vi "deleteDesFromEEPROMFiles.vi"(11 "input_eeprom":string[][](array[string])) -> (3 "show_eeprom":string[][](array[string]))   [LabVIEW 2011]
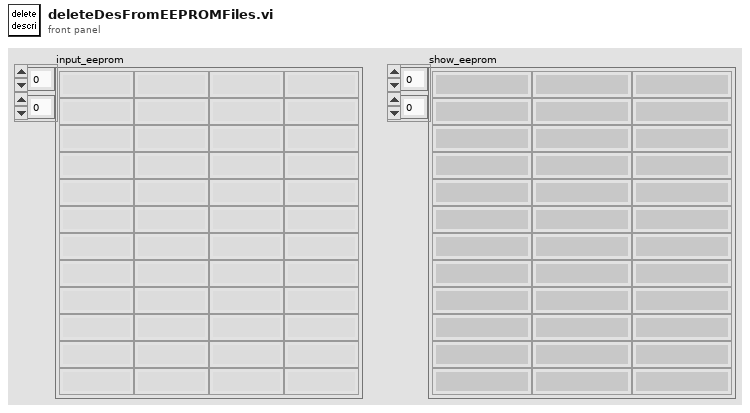
[diagram p1: front panel]
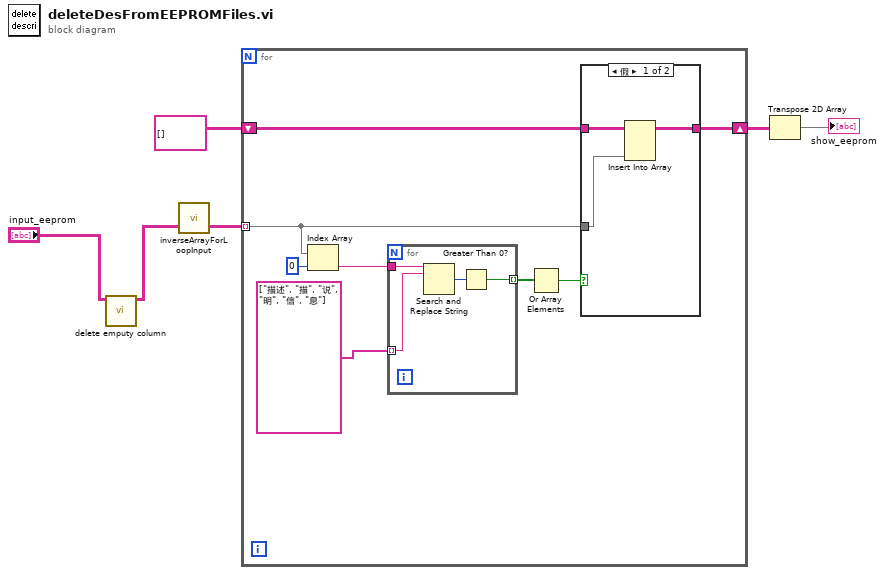
[diagram p0: block diagram]
diagram:
  n1 = call "delete emputy column.vi"("input_eeprom"="input_eeprom") -> ("input_eeprom_deleteemputycolumn"=w1:string[][])  [unwired: 10 in]
  n2 = call "inverseArrayForLoopInput.vi"("input_array_temp_str"=w1) -> ("show_array_temp_str"=w6:string[][])  [unwired: 1 in, 1 out]
  n3 = for {
    tunnel: w6 -> [w8] mode=indexing
    shift-right: [w7] -> w4
    shift-left: string[][] [] -> [w9]
    n4 = Index Array(array=w8, index=0 ("索引")) -> (element=w12:string)
    n5 = for {
      tunnel: string[] ["描述", "描", "说", "明", "信", "息"] -> [w21] mode=indexing
      tunnel: w12 -> [w22]
      tunnel: [w19] -> w11 mode=indexing
      n6 = Search and Replace String(input string=w22, search string=w21) -> (number of replacements=w20:i32)  [unwired: 6 in, 3 out]
      n7 = Greater Than 0?(x=w20) -> (x > 0?=w19:bool)
    }
    n8 = Or Array Elements(Boolean array=w11) -> (logical OR=w10:bool)
    n9 = case shown="假" w10 {
      tunnel: w9 -> [w17 w18]
      tunnel: w8 -> [w16 _]
      tunnel: [w15 w18] -> w7
      frame False {
        n10 = Insert Into Array(array=w17, new element=w16) -> (w15:string[][])  [unwired: 2 in]
      }
      frame True {
      }
    }
  }
  n11 = Transpose 2D Array(2D array=w4) -> (transposed array=→"show_eeprom":string[][])
